vi "S2DS_Ramp or Go to (SubVI).vi"(11 "Scan parameters in":T1 {"Y data taking" items=["in both direction", "in up direction only", "in down direction only"]; "X data taking" items=["in both direction", "in up direction only", "in down direction only"]}) -> (3 "Scan parameters out":T1 {"Y data taking" items=["in both direction", "in up direction only", "in down direction only"]; "X data taking" items=["in both direction", "in up direction only", "in down direction only"]})   [LabVIEW 2025]
uses:
  TYPE DEFS/S2DS_Sweep Info.ctl
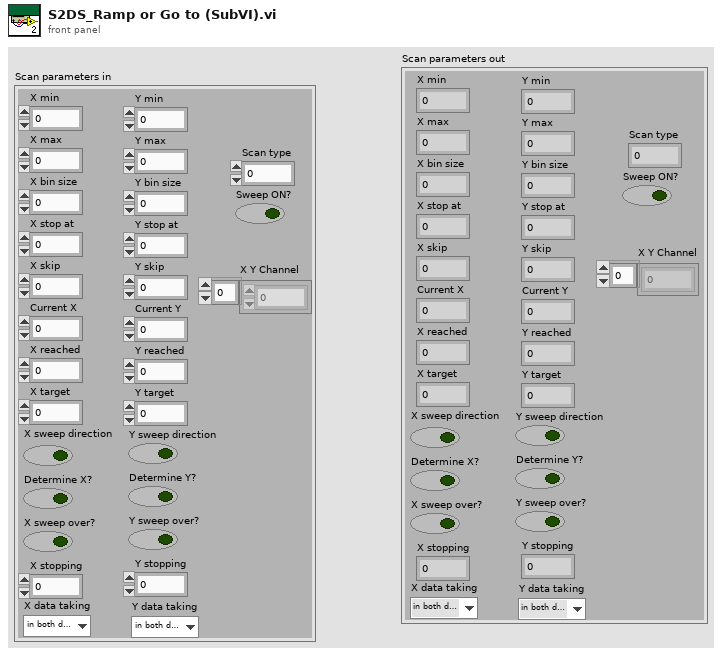
[diagram p1: front panel]
types:
  T1 = typedef "S2DS_Sweep Info.ctl" = cluster{"X min":ext, "X max":dbl, "Y min":dbl, "Y max":dbl, "X bin size":dbl, "Y bin size":dbl, "X stop at":dbl, "Y stop at":dbl, "X skip":u64, "Y skip":u64, "Current X":dbl, "Current Y":dbl, "X reached":i32, "Y reached":i32, "X target":dbl, "Y target":dbl, "Sweep ON?":bool, "X sweep direction":bool, "Y sweep direction":bool, "Determine X?":bool, "Determine Y?":bool, "X sweep over?":bool, "Y sweep over?":bool, "Scan type":i32, "X stopping":i32, "Y stopping":i32, "X Y Channel":u16[], "X data taking":u16, "Y data taking":u16}
  T2 = enum16{"Left Button", "Center Button", "Right Button", "Window Close"}
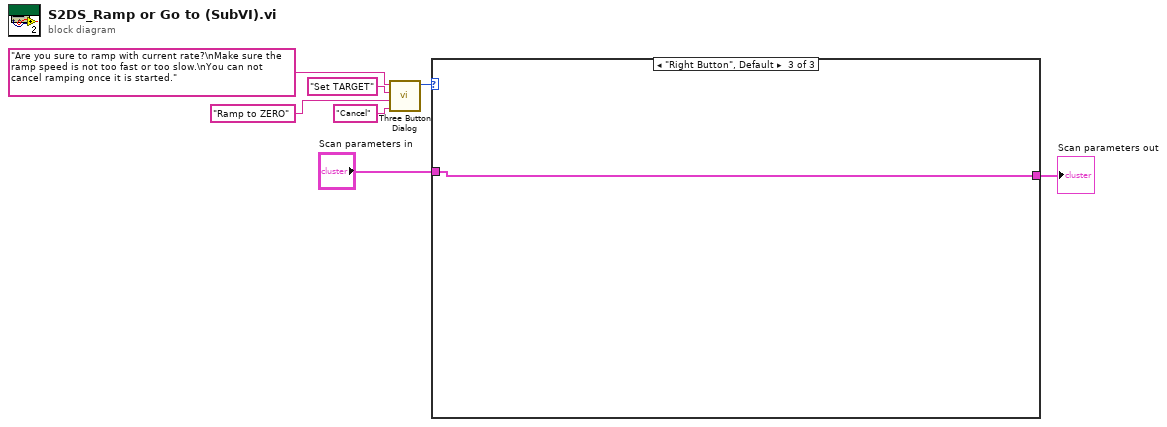
[diagram p0: block diagram]
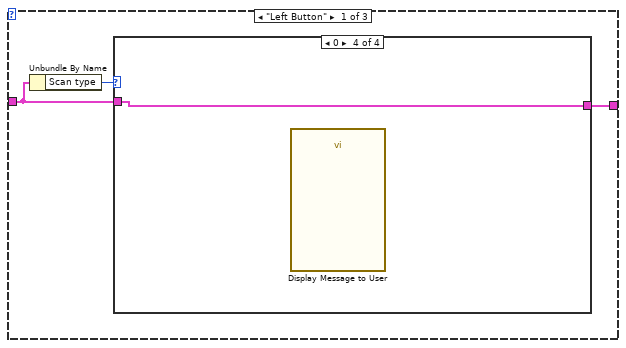
[diagram p2: hidden frame]
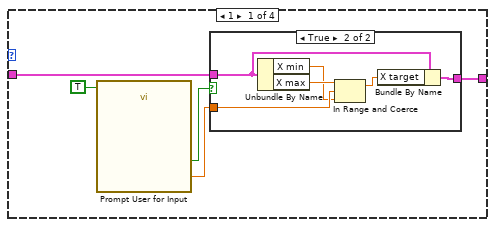
[diagram p3: hidden frame]
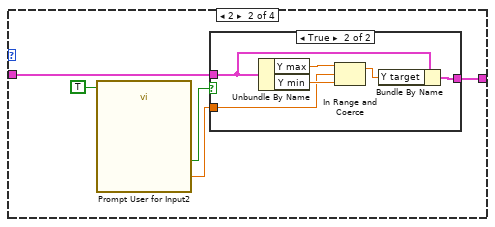
[diagram p5: hidden frame]
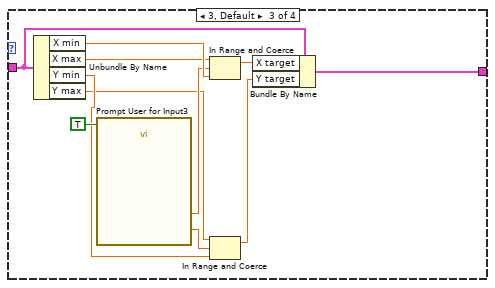
[diagram p7: hidden frame]
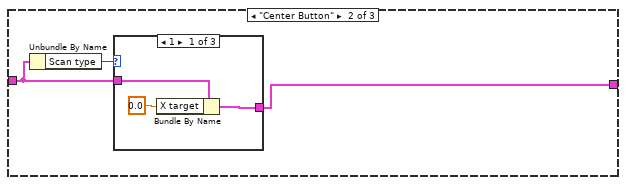
[diagram p8: hidden frame]
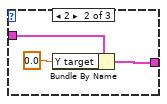
[diagram p9: hidden frame]
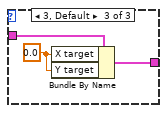
[diagram p10: hidden frame]
diagram:
  n1 = call <vilib>:"Three Button Dialog.vi"("Right Button Text (\"Cancel\")"="Cancel" ("Right Button Text (\"Cancel\")"), "Center Button Text (\"No\")"="Ramp to ZERO" ("Center Button Text (\"No\")"), "Left Button Text (\"Yes\")"="Set TARGET" ("Left Button Text (\"Yes\")"), "message"="Are you sure to ramp with current rate?\nMake sure the ramp speed is not too fast or too slow.\nYou can not cancel ramping once it is started.") -> ("Which Button?"=w4:T2)  [unwired: 7 in]
  n2 = case shown="\"Right Button\", Default" w4 {
    tunnel: "Scan parameters in" -> [w9 w48 w59]
    tunnel: [w8 w49 w59] -> w7
    frame "Left Button" {
      n3 = Unbundle By Name(w9) -> ("Scan type"=w10:i32)
      n4 = case shown="0" w10 {
        tunnel: [w12 w24 w45 w46] -> w8
        tunnel: w9 -> [w13 w25 w43 w46]
        frame 1 {
          n5 = call "Prompt User for Input"("Enable"=TRUE) -> ("X target"=w11:dbl, "OK"=w14:bool)  [unwired: 16 in, 1 out]
          n6 = case shown="True" w14 {
            tunnel: w13 -> [w16 w20]
            tunnel: [w16 w22] -> w12
            tunnel: w11 -> [_ w21]
            frame False {
            }
            frame True {
              n7 = Unbundle By Name(w20) -> ("X min"=w18:ext, "X max"=w19:dbl)
              n8 = In Range and Coerce(upper limit=w19, x=w21, lower limit=w18) -> (coerced(x)=w17:ext)  [unwired: 1 out]
              n9 = Bundle By Name(cluster=w20, "X target"=w17) -> (w22:T1)
            }
          }
        }
        frame 2 {
          n10 = call "Prompt User for Input2"("Enable"=TRUE) -> ("Y target"=w23:dbl, "Ramp"=w26:bool)  [unwired: 16 in, 1 out]
          n11 = case shown="True" w26 {
            tunnel: w25 -> [w28 w33]
            tunnel: [w28 w34] -> w24
            tunnel: w23 -> [_ w30]
            frame False {
            }
            frame True {
              n12 = Unbundle By Name(w33) -> ("Y max"=w32:dbl, "Y min"=w31:dbl)
              n13 = In Range and Coerce(upper limit=w32, x=w30, lower limit=w31) -> (coerced(x)=w29:dbl)  [unwired: 1 out]
              n14 = Bundle By Name(cluster=w33, "Y target"=w29) -> (w34:T1)
            }
          }
        }
        frame 3, Default {
          n15 = Unbundle By Name(w43) -> ("X min"=w42:ext, "X max"=w41:dbl, "Y min"=w39:dbl, "Y max"=w38:dbl)
          n16 = call "Prompt User for Input3"("Enable"=TRUE) -> ("Y target"=w37:dbl, "X target"=w40:dbl)  [unwired: 15 in, 2 out]
          n17 = In Range and Coerce(upper limit=w41, x=w40, lower limit=w42) -> (coerced(x)=w36:ext)  [unwired: 1 out]
          n18 = In Range and Coerce(upper limit=w38, x=w37, lower limit=w39) -> (coerced(x)=w35:dbl)  [unwired: 1 out]
          n19 = Bundle By Name(cluster=w43, "X target"=w36, "Y target"=w35) -> (w45:T1)
        }
        frame 0 {
          n20 = call "Display Message to User"() -> ()  [unwired: 10 in, 2 out]
        }
      }
    }
    frame "Center Button" {
      n21 = Unbundle By Name(w48) -> ("Scan type"=w47:i32)
      n22 = case shown="1" w47 {
        tunnel: [w51 w54 w57] -> w49
        tunnel: w48 -> [w52 w55 w58]
        frame 1 {
          n23 = Bundle By Name(cluster=w52, "X target"=0.0) -> (w51:T1)
        }
        frame 2 {
          n24 = Bundle By Name(cluster=w55, "Y target"=0.0) -> (w54:T1)
        }
        frame 3, Default {
          w56 = 0.0 ("Y target")
          n25 = Bundle By Name(cluster=w58, "X target"=w56, "Y target"=w56) -> (w57:T1)
        }
      }
    }
    frame "Right Button", Default {
    }
  }
  "Scan parameters out" <- w7
